vi "Append a Picture.vi"(8 "error in (no error)":errorcluster, 10 "Picture File Path":path, 11 "xwpfParagraph in":refnum<class "xwpfParagraph.lvclass">) -> (0 "error out":errorcluster, 3 "xwpfParagraph out":refnum<class "xwpfParagraph.lvclass">)   [LabVIEW 2017, in "Word_Specific.lvlib" / "xwpfParagraph.lvclass"]
uses:
  xwpfParagraph.lvclass
  xwpfRun.Figure/xwpfRun.Figure.lvclass
  C:/Users/Neo/Desktop/Dev_Tools_BR/LabVIEW_NPOI/src/LabVIEW NPOI/xwpfRun/xwpfRun.lvclass
  xwpfParagraph.lvclass/xwpfParagraph.ctl
  C:/Users/Neo/Desktop/Dev_Tools_BR/LabVIEW_NPOI/lib/NPOI 2.1.1/NPOI.OOXML.dll
  lib/NPOI 2.1.1/NPOI.OOXML.dll
  xwpfRun.Figure/xwpfRun.Figure.lvclass/xwpfRun.Figure.ctl
  xwpfRun.Figure/Set Picture.File Path.vi
  xwpfRun/xwpfRun.lvclass
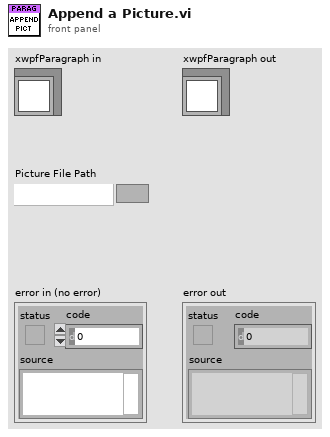
[diagram p1: front panel]
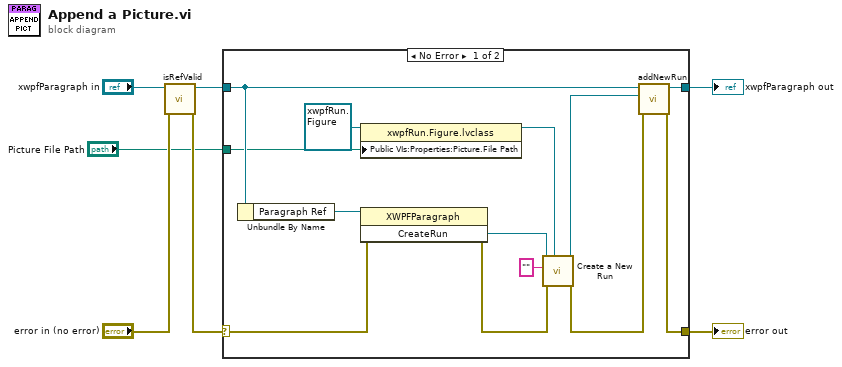
[diagram p0: block diagram]
diagram:
  n1 = call-dynamic "isRefValid.vi"("error in (no error)"="error in (no error)", "xwpfParagraph in"="xwpfParagraph in") -> ("error out"=w2:errorcluster, "xwpfParagraph out"=w4:refnum<class "xwpfParagraph.lvclass">)  [unwired: 8 in]
  n2 = case shown="No Error" w2 {
    selector: w2 -> [w12 w22]
    tunnel: [w14 w22] -> w7
    tunnel: [w17 w21] -> w5
    tunnel: w4 -> [w13 w21]
    tunnel: "Picture File Path" -> [w8 _]
    frame No Error {
      n3 = Unbundle By Name(w13) -> ("Paragraph Ref"=w20:refnum<k24>)
      n4 = property class="xwpfRun.Figure.lvclass"(reference=refnum<class "xwpfRun.Figure.lvclass"> refnum ("xwpfRun.Figure in"), "Public VIs:Properties:Picture.File Path"=w8) -> (reference out=w9:refnum<class "xwpfRun.Figure.lvclass">)  [unwired: 1 in, 1 out]
      n5 = invoke class="XWPFParagraph" method="CreateRun"(reference=w20, error in=w12) -> (error out=w18:errorcluster, "CreateRun"=w19:refnum<k24>)  [unwired: 1 in, 1 out]
      n6 = call "Create a New Run.vi"("xwpfRun Type"=w9, "error in (no error)"=w18, "Text"="", "Run Ref"=w19) -> ("error out"=w15:errorcluster, "xwpfRun out"=w16:refnum<class "xwpfRun.Figure.lvclass">)  [unwired: 6 in]
      n7 = call "addNewRun.vi"("error in (no error)"=w15, "New Run"=w16, "xwpfParagraph in"=w13) -> ("error out"=w14:errorcluster, "xwpfParagraph out"=w17:refnum<class "xwpfParagraph.lvclass">)  [unwired: 7 in]
    }
    frame Error {
    }
  }
  "error out" <- w7
  "xwpfParagraph out" <- w5
